vi "Calc - Pamb P.vi"(11 "00-00-9220":dbl[](array[numeric])) -> (3 "Pamb P":dbl)   [LabVIEW 2018, in "Controller (Host).lvlib"]
uses:
  Controller (Host).lvlib
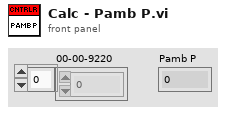
[diagram p1: front panel]
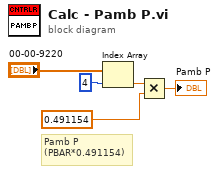
[diagram p0: block diagram]
diagram:
  # "Pamb P\n(PBAR*0.491154)"
  n1 = Index Array(array="00-00-9220", index=4) -> (element=w1:dbl)
  n2 = Multiply(x=w1, y=0.491154) -> (x*y=→"Pamb P":dbl)
